vi "CALC_RDATA.vi"(0 "VISA IN":refnum<visa-resource-name>, 1 "Physical Receiver":string, 5 "error in":errorcluster, 7 "Channel":i32) -> (14 "VISA Out":refnum<visa-resource-name>, 16 "Data":string, 19 "error out":errorcluster)   [LabVIEW 2018, in "PNA-X.lvlib"]
doc: "CALCulate<cnum>:RDATA? <char> \n(Read-only) Returns receiver data for the selected measurement. To query measurement data, see \nCALC:DATA? \nParameters \n<cnum> Channel number of the measurement. There must be a selected measurement \non that channel. If unspecified, <cnum> is set to 1. \n<char> Choose from any physical receiver in the PNA. \nFor example: \"A\" \nAlso, REF - returns data for either R1 or R2 data depending on the source port \nof the selected measurement. \nSee the block diagram showing the receivers in YOUR PNA. \nNote: Logical receiver notation is NOT allowed with this command. Learn \nmore. \nExample GPIB.Write \"INITiate:CONTinuous OFF\" \nGPIB.Write \"INITiate:IMMediate;*wai\" \nGPIB.Write \"CALCulate:RDATA? A\" \nGPIB.Write \"CALCulate:RDATA? REF\" \nReturn Type Depends on FORM:DATA - Two numbers per data point \nDefault Not Applicable \nNotes: \nGenerally when you query the analyzer for data, you expect that the number of data values returned will \nbe consistent with the number of points in the sweep. \nHowever, if you query receiver data while the instrument is sweeping, the returned values may contain \nzeros. For example, if your request for receiver data is handled on the 45th point of a 201 point sweep, \nthe first 45 values will be valid data, and the remainder will contain complex zero. \nThis can be avoided by synchronizing this request with the end of a sweep or putting the channel in \nhold mode. \n1561\n\nLearn about Unratioed Measurements \n1562\n\nCalculate:Smoothing Commands \nControls point-to-point smoothing. Smoothing is a noise reduction technique that averages adjacent \ndata points in a measurement trace. Choose the amount of smoothing by specifying either the number \nof points or the aperture. Smoothing is not the same as CALC:AVERage which averages each data \npoint over a number of sweeps. \nClick on a blue keyword to view the command details. \nSee Also \nExample Programs \nLearn about Smoothing \nSynchronizing the PNA and Controller \nSCPI Command Tree \nCritical Note: CALCulate commands act on the selected measurement. You can select one \nmeasurement for each channel using Calc:Par:Select"
uses:
  PNA-X.lvlib
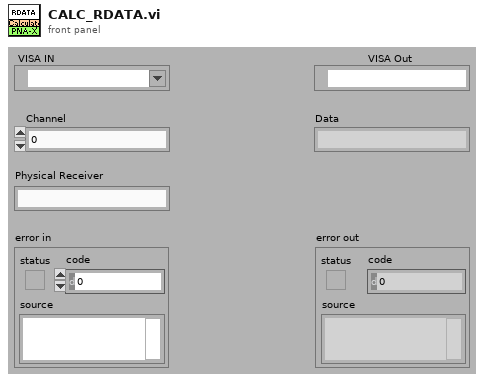
[diagram p1: front panel]
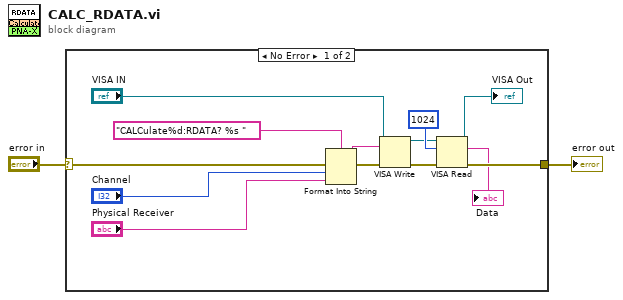
[diagram p0: block diagram]
diagram:
  n1 = case shown="No Error" "error in" {
    selector: "error in" -> [w15 w16]
    tunnel: [w7 w16] -> w1
    frame No Error {
      n2 = Format Into String(format string="CALCulate%d:RDATA? %s " ("Cmdline"), error in=w15, "Channel", "Physical Receiver") -> (resulting string=w13:string, error out=w14:errorcluster)  [unwired: 1 in]
      n3 = VISA Write(VISA resource name="VISA IN", write buffer=w13, error in (no error)=w14) -> (VISA resource name out=w8:refnum<visa-resource-name>, error out=w10:errorcluster)  [unwired: 1 out]
      n4 = VISA Read(VISA resource name=w8, byte count=1024, error in (no error)=w10) -> (VISA resource name out=→"VISA Out":refnum<visa-resource-name>, read buffer=→"Data":string, error out=w7:errorcluster)  [unwired: 1 out]
    }
    frame Error {
    }
  }
  "error out" <- w1
